vi "Init Arrduino.vi"(2 "error in (no error)":errorcluster, 3 "baud rate (9600)":u32=9600, 4 "VISA Refnum in":refnum<visa-resource-name>) -> (0 "error out":errorcluster, 1 "VISA Refnum out":refnum<visa-resource-name>)   [LabVIEW 2014]
uses:
  <vilib>/Instr/_visa.llb/VISA Configure Serial Port (Instr).vi
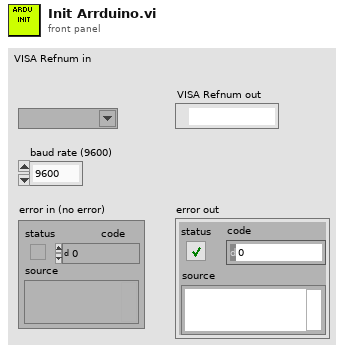
[diagram p1: front panel]
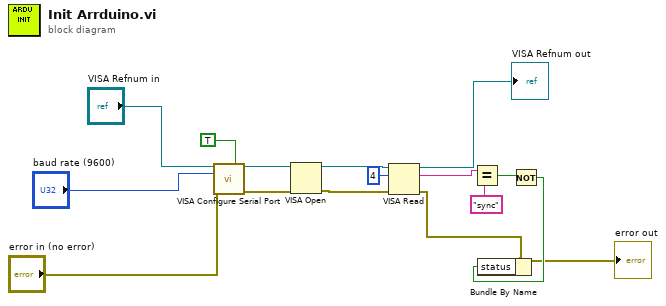
[diagram p0: block diagram]
diagram:
  n1 = call-poly "VISA Configure Serial Port"("VISA resource name"="VISA Refnum in", "Enable Termination\nChar (T)"=TRUE ("Enable Termination\nChar (T)"), "baud rate (9600)"="baud rate (9600)", "error in (no error)"="error in (no error)") -> ("VISA resource name out"=w4:refnum<visa-resource-name>, "error out"=w5:errorcluster)  [unwired: 10 in]
  n2 = VISA Open(error in (no error)=w5, VISA resource name=w4) -> (VISA resource name=w6:refnum<visa-resource-name>, error out=w7:errorcluster)  [unwired: 3 in]
  n3 = VISA Read(VISA resource name=w6, byte count=u32 4, error in (no error)=w7) -> (VISA resource name out=→"VISA Refnum out":refnum<visa-resource-name>, read buffer=w9:string, error out=w11:errorcluster)  [unwired: 1 out]
  "error out" <- w11
  n4 = Equal?(x=w9, y="sync") -> (x = y?=w12:bool)
  n5 = Not(x=w12) -> (.not. x?=w13:bool)
  n6 = Bundle By Name(cluster=w11, "status"=w13) -> ()  [unwired: 1 out]
